vi "Get Value From DVR Ref TEST.vi"() -> ()   [LabVIEW 2018]
uses:
  class1/TypeDef/Data.ctl
  class1/TypeDef/Settings.ctl
  <vilib>/Utility/miscctls.llb/LVPointTypeDef.ctl
  34080777-38a0-4f01-a48f-5d341e4b3cf4.vi
  class1/class1.lvclass
  <vilib>/Utility/Data Type/NI_Data Type.lvlib
panel:
  out "data value 2":cluster{i32, string}
  out "Controls[]":refnum<vi>[](array[refnum])
  out "data value reference":refnum<data-value>
  out "Array":string[](array[string])
  out "Cluster Elements":variant[](array[variant])
  out "error out":errorcluster
  in  "DVR":refnum<data-value>
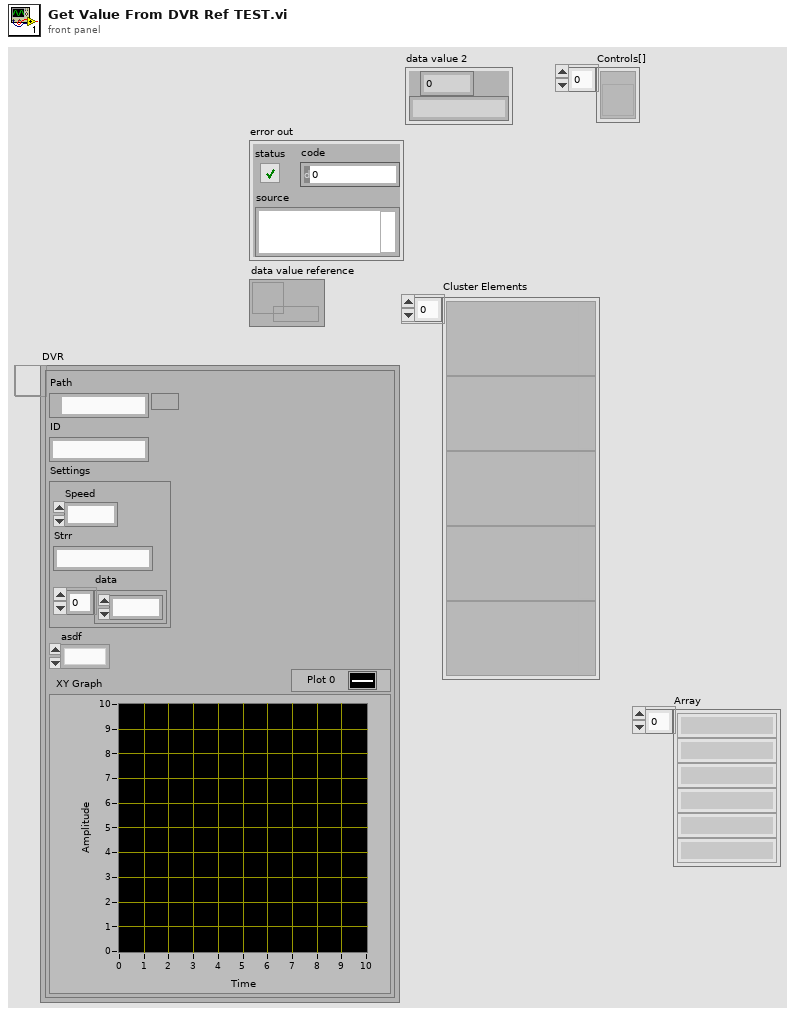
[diagram p1: front panel]
types:
  T1 = enum8{"Probe", "Diagram", "Panel Control", "3D Panel Control", "Dialog Panel Control", "Panel Indicator", "3D Panel Indicator", "Dialog Panel Indicator", "Power PC Control", "Power PC Indicator", "Silver Control", "Silver Indicator", "NXG Style Control", "NXG Style Indicator"}
  T2 = typedef "LVPointTypeDef.ctl" = cluster{"Horizontal":i16, "Vertical":i16}
  T3 = typedef "class1.lvclass/Data.ctl" = cluster{"Path":path, "ID":string, "Settings":T4, "asdf":enum16{"a", "f"}, "XY Graph":cluster{"X":dbl, "Y":dbl}[]}
  T4 = typedef "class1.lvclass/Settings.ctl" = cluster{"Speed":dbl, "Strr":string, "data":i32[]}
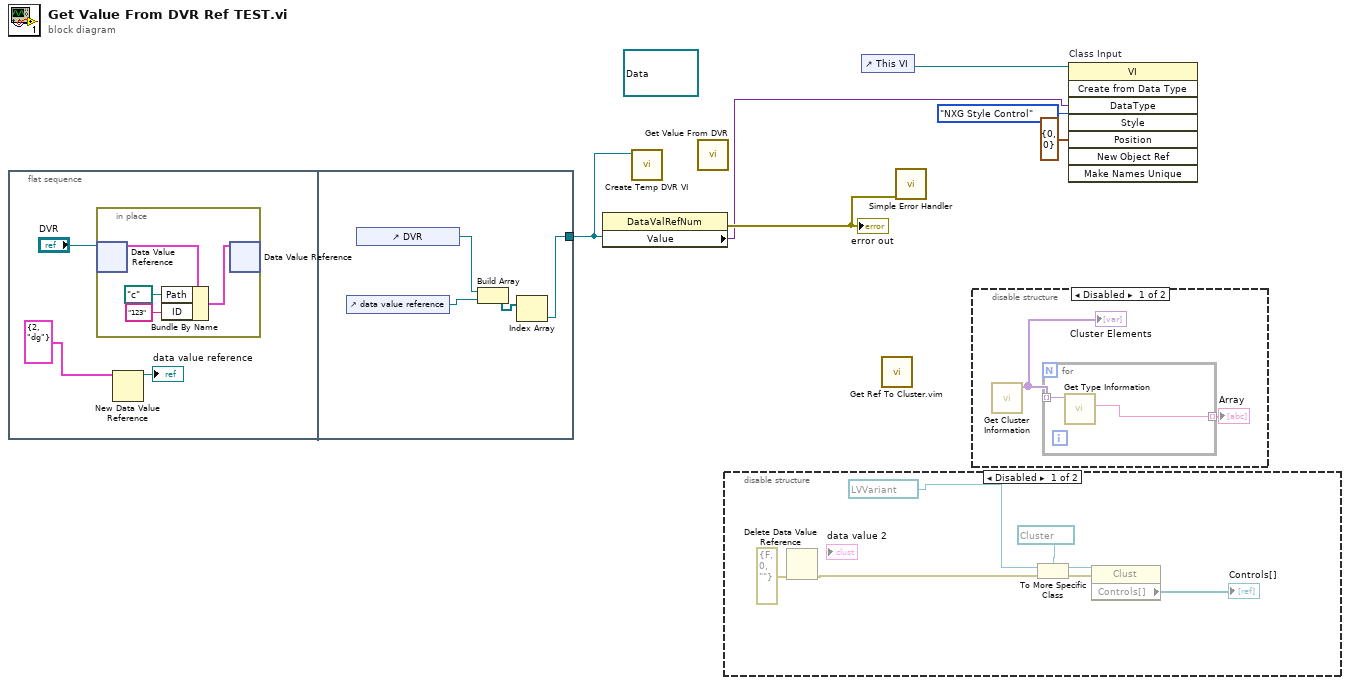
[diagram p0: block diagram]
diagram:
  (unwired) refnum<data-value> refnum ("DVR")
  n1 = flat-sequence {
    tunnel: [w14] -> w1
    frame #0 {
      n2 = in-place {
        n3 = in-place-dvr #1("DVR") -> (w13:T3)  [unwired: 1 out]
        n4 = Bundle By Name(cluster=w13, "Path"=path "c:/", "ID"="123") -> (w12:T3)
        n5 = in-place-dvr #1(w12) -> ()  [unwired: 2 out]
      }
      n6 = New Data Value Reference(data value=cluster{i32, string} {2, "dg"}) -> (data value reference=→"data value reference":refnum<data-value>)  [unwired: 1 in, 1 out]
    }
    frame #1 {
      n7 = control-ref of="data value reference"() -> (w17:refnum<vi>)
      n8 = control-ref of="DVR"() -> (w15:refnum<vi>)
      n9 = Build Array(w15, w17) -> (w16:refnum<vi>[])
      n10 = Index Array(array=w16) -> (element=w14:refnum<vi>)  [unwired: 1 in]
    }
  }
  n11 = property class="DataValRefNum"(reference=w1) -> (error out=w6:errorcluster, "Value"=w2:variant)  [unwired: 1 in, 1 out]
  "error out" <- w6
  n12 = call "Create Temp DVR VI.vi"("DataValRefNum in"=w1) -> ()  [unwired: 10 in, 1 out]
  n13 = call "Get Value From DVR.vi"() -> ()  [unwired: 10 in, 2 out]
  n14 = disable-structure shown="Disabled" {
    frame Disabled {
      n15 = Delete Data Value Reference(error in=errorcluster {"status"=FALSE, "code"=0, "source"=""} ("error in (no error)")) -> (data value reference=w18:refnum<data-value>, error out=w24:errorcluster)  [unwired: 1 out]
      n16 = To More Specific Class(target class=refnum<vi> refnum ("DVR"), reference=refnum<vi> refnum ("Element.Value 2"), error in=w24) -> (specific class reference=w23:refnum<vi>, error out=w22:errorcluster)
      n17 = property class="Clust"(reference=w23, error in=w22) -> ("Controls[]"=→"Controls[]":refnum<vi>[])  [unwired: 2 out]
    }
    frame Enabled {
    }
  }
  n18 = control-ref of="This VI"() -> (w5:refnum<vi>)
  n19 = call "Get Ref To Cluster.vim"() -> ()  [unwired: 11 in, 1 out]
  n20 = call <vilib>:"Simple Error Handler.vi"("error in (no error)"=w6) -> ()  [unwired: 4 in, 5 out]
  n21 = disable-structure shown="Disabled" {
    frame Disabled {
      n22 = call <vilib>:"Get Cluster Information.vi"() -> ("Cluster Elements"=w27:variant[])  [unwired: 10 in, 1 out]
      "Cluster Elements" <- w27
      n23 = for {
        tunnel: w27 -> [w29] mode=indexing
        tunnel: [w28] -> w26 mode=indexing
        n24 = call <vilib>:"Get Type Information.vi"("Variant"=w29) -> ("Name"=w28:string)  [unwired: 6 in, 4 out]
      }
      "Array" <- w26
    }
    frame Enabled {
    }
  }
  n25 = invoke on="Class Input" class="VI" method="Create from Data Type"(reference=w5, "DataType"=w2, "Style"=T1."NXG Style Control", "Position"=T2 {"Horizontal"=0, "Vertical"=0}) -> ()  [unwired: 4 in, 8 out]
